vi "Configure Event Callback.vi"(8 "error in (no error)":errorcluster) -> (0 "error out":errorcluster)   [LabVIEW 2025]
uses:
  Control Globals.vi
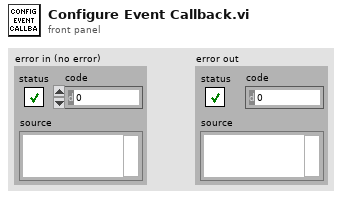
[diagram p1: front panel]
types:
  T1 = cluster{"Top level VI":refnum<vi>, "ExecutionView Manager":refnum<k7>}
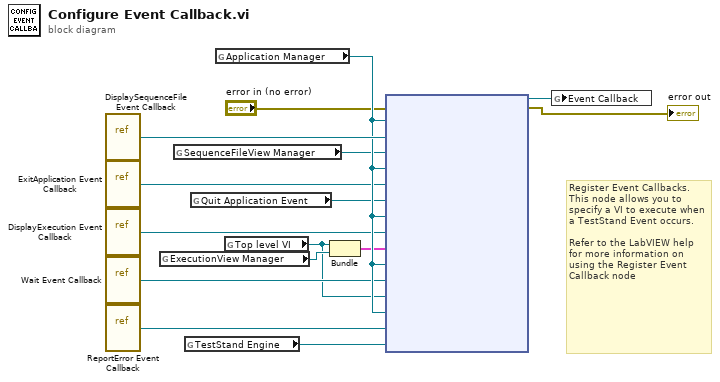
[diagram p0: block diagram]
diagram:
  # "Register Event Callbacks.  This node allows you to specify a VI to execute when a TestStand Event occurs. \n\nRefer to the LabVIEW help for more information on using the Register Event Callback node"
  n1 = vi-ref "DisplaySequenceFile Event Callback.vi"() -> ("vi reference"=w15:refnum<vi>)
  n2 = vi-ref "ExitApplication Event Callback.vi"() -> ("vi reference"=w12:refnum<vi>)
  n3 = vi-ref "DisplayExecution Event Callback.vi"() -> ("vi reference"=w10:refnum<vi>)
  n4 = vi-ref "Wait Event Callback.vi"() -> ("vi reference"=w9:refnum<vi>)
  n5 = vi-ref "ReportError Event Callback.vi"() -> ("vi reference"=w11:refnum<vi>)
  n6 = global read "Control Globals.vi" "ExecutionView Manager"() -> (w4:refnum<k7>)
  n7 = global read "Control Globals.vi" "SequenceFileView Manager"() -> (w6:refnum<k7>)
  n8 = global read "Control Globals.vi" "TestStand Engine"() -> (w1:refnum<k7>)
  n9 = global read "Control Globals.vi" "Quit Application Event"() -> (w5:refnum<user-event>)
  n10 = global read "Control Globals.vi" "Application Manager"() -> (w14:refnum<k7>)
  n11 = global read "Control Globals.vi" "Top level VI"() -> (w2:refnum<vi>)
  n12 = Bundle("Top level VI"=w2, "ExecutionView Manager"=w4) -> (w3:T1)  [unwired: 1 in]
  n13 = node("error in (no error)", w14, w15, w6, w14, w12, w5, w14, w10, w3, w14, w9, w2, w14, w11, w1) -> (w13:refnum<k27>, →"error out":errorcluster)  [unwired: 1 in]
  n14 = global write "Control Globals.vi" "Event Callback"(w13) -> ()
